vi "deleteStaleSqliteData.vi"() -> ()   [LabVIEW 2023]
uses:
  <vilib>/drjdpowell/SQLite Library/SQL Connection/Connection.lvclass
  <vilib>/drjdpowell/SQLite Library/SQL Connection/Open (path).vi
  <vilib>/drjdpowell/SQLite Library/SQLite.lvlib
  <vilib>/drjdpowell/SQLite Library/SQL Connection/Execute SQL (No results).vi
  <vilib>/drjdpowell/SQLite Library/SQL Statement/SQL Statement.lvclass
  <vilib>/drjdpowell/SQLite Library/Transaction Helpers/Transaction.lvlib
panel:
  in  "Path to local database file *.db":path=path "C:/sqlite/sensor_data.db"
  out "Rows (Samples) Detected in input array":i32=1000
  in  "Savepoint name":string="MySavepoint"
  in  "SQLite Command":string="CREATE TABLE IF NOT EXISTS pipe_data(\nID INTEGER PRIMARY KEY AUTOINCREMENT,\nUNIX_TIME REAL NOT NULL, \nPRESSURE REAL NOT NULL,\nTEMPERATURE REAL NOT NULL,\nDENSITY REAL NOT NULL\n);"
  in  "error in (no error)":errorcluster
  out "error out":errorcluster
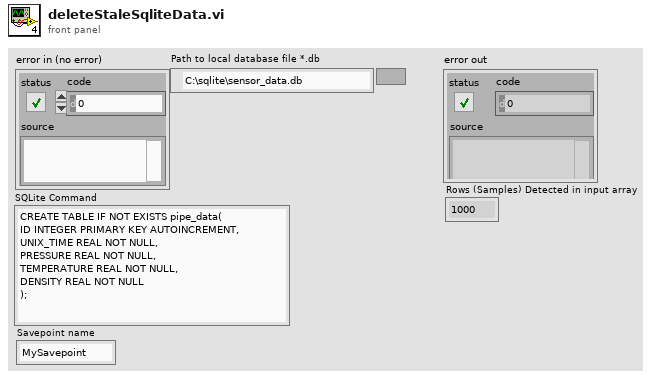
[diagram p1: front panel]
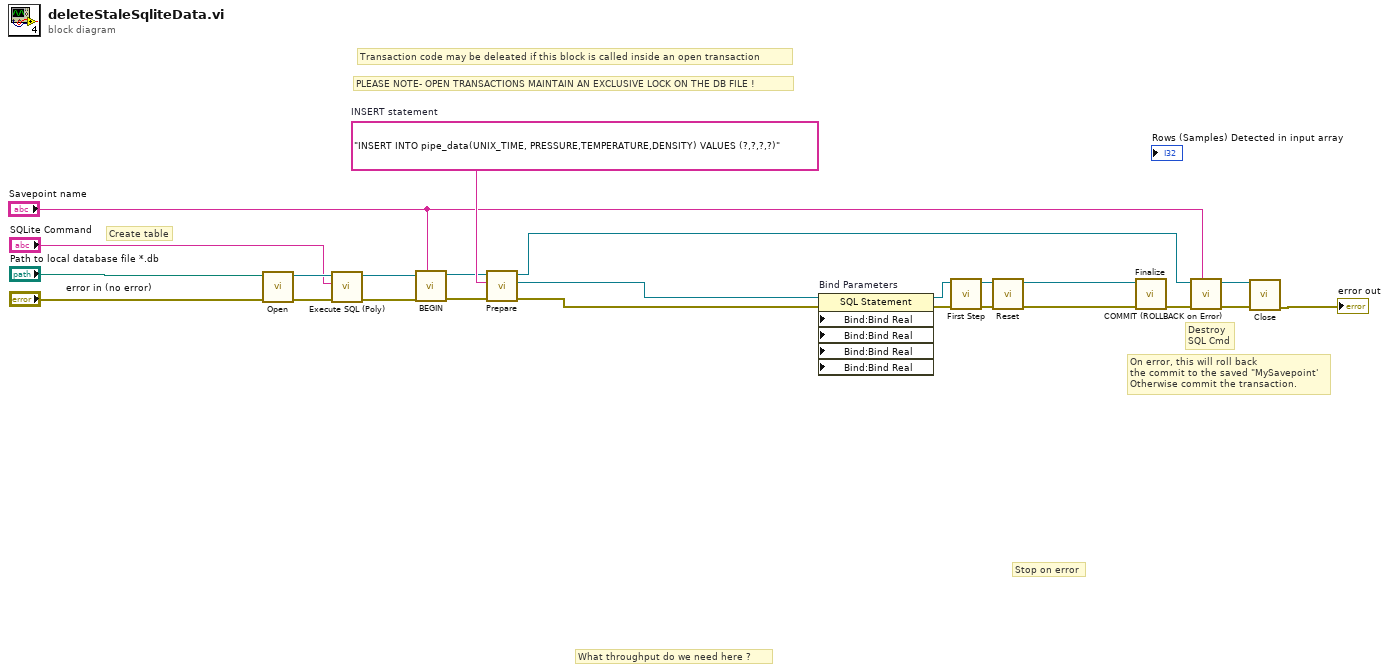
[diagram p0: block diagram]
diagram:
  w14 = "INSERT INTO pipe_data(UNIX_TIME, PRESSURE,TEMPERATURE,DENSITY) VALUES (?,?,?,?)"  # INSERT statement
  # "Stop on error"
  # "What throughput do we need here ?"
  # "Create table"
  # "Destroy\nSQL Cmd"
  # "On error, this will roll back\nthe commit to the saved \"MySavepoint'\nOtherwise commit the transaction."
  # "PLEASE NOTE- OPEN TRANSACTIONS MAINTAIN AN EXCLUSIVE LOCK ON THE DB FILE !"
  # "Transaction code may be deleated if this block is called inside an open transaction"
  n1 = call-poly <vilib>:"Open.vi"("error in (no error)"="error in (no error)", "db file"="Path to local database file *.db") -> ("error out"=w6:errorcluster, "SQLite Connection"=w18:refnum<class "Connection.lvclass">)  [unwired: 8 in]
  n2 = call-poly <vilib>:"Execute SQL (Poly).vi"("error in (no error)"=w6, "SQL"="SQLite Command", "SQLite Connection in"=w18) -> ("error out"=w16:errorcluster, "SQLite Connection"=w19:refnum<class "Connection.lvclass">)  [unwired: 7 in]
  n3 = call <vilib>:"BEGIN.vi"("Savepoint name"="Savepoint name", "error in (no error)"=w16, "SQLite Connection in"=w19) -> ("error out"=w10:errorcluster, "SQLite Connection"=w11:refnum<class "Connection.lvclass">)  [unwired: 7 in]
  n4 = call <vilib>:"Prepare.vi"("error in (no error)"=w10, "SQL"=w14, "SQLite Connection in"=w11) -> ("error out"=w23:errorcluster, "SQL Statement"=w15:refnum<class "SQL Statement.lvclass">, "SQLite Connection"=w8:refnum<class "Connection.lvclass">)  [unwired: 4 in, 2 out]
  n5 = property on="Bind Parameters" class="SQL Statement" props=["Bind:Bind Real", "Bind:Bind Real", "Bind:Bind Real", "Bind:Bind Real"](reference=w15, error in=w23) -> (reference out=w4:refnum<class "SQL Statement.lvclass">, error out=w3:errorcluster)  [unwired: 4 in]
  n6 = call <vilib>:"First Step.vi"("error in (no error)"=w3, "SQL Statement in"=w4) -> ("error out"=w2:errorcluster, "SQL Statement"=w1:refnum<class "SQL Statement.lvclass">)  [unwired: 7 in, 1 out]
  n7 = call <vilib>:"Reset.vi"("error in (no error)"=w2, "SQL Statement in"=w1) -> ("error out"=w12:errorcluster, "SQL Statement"=w13:refnum<class "SQL Statement.lvclass">)  [unwired: 8 in]
  n8 = call <vilib>:"Finalize.vi"("error in (no error)"=w12, "SQL Statement in"=w13) -> ("error out"=w7:errorcluster)  [unwired: 9 in]
  n9 = call <vilib>:"COMMIT (ROLLBACK on Error).vi"("Savepoint name"="Savepoint name", "error in (no error)"=w7, "SQLite Connection in"=w8) -> ("error out"=w22:errorcluster, "SQLite Connection"=w21:refnum<class "Connection.lvclass">)  [unwired: 7 in]
  n10 = call-dynamic "Close.vi"("error in (no error)"=w22, "SQLite Connection in"=w21) -> ("error out"=→"error out":errorcluster)  [unwired: 9 in]
